vi "Connect.vi"(8 "error in":errorcluster, 11 "2727 in":refnum<class "2727.lvclass">) -> (0 "error out":errorcluster, 3 "2727 out":refnum<class "2727.lvclass">)   [LabVIEW 2019, in "2727.lvlib" / "2727.lvclass"]
uses:
  Library/2727.lvclass
  C:/Users/Public/Documents/Development/builds/Instruments/Instruments.lvlibp/Library/Instruments.lvclass
  Library/2727.lvclass/2727.ctl
  builds/Instruments/Instruments.lvlibp/Accessors/Read Resource.vi
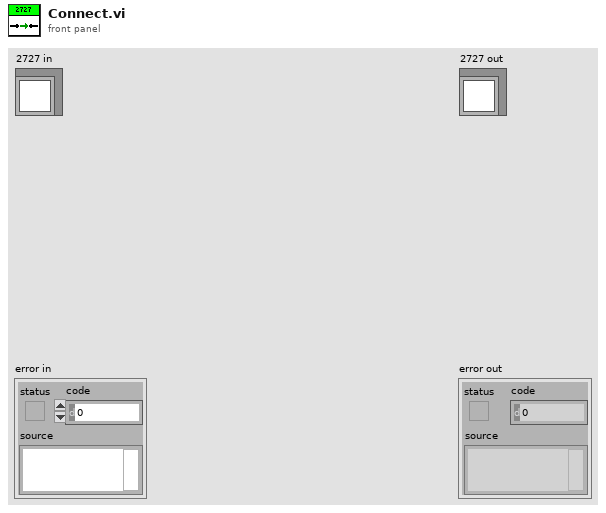
[diagram p1: front panel]
types:
  T1 = typedef "ni272x Reference.ctl" = refnum<k20>
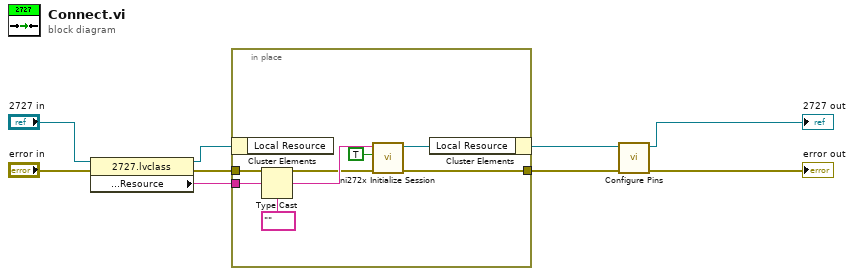
[diagram p0: block diagram]
diagram:
  n1 = property class="2727.lvclass"(reference="2727 in", error in="error in") -> (reference out=w6:refnum<class "2727.lvclass">, error out=w8:errorcluster, "Accessors:Configuration:Resource"=w5:string)
  n2 = in-place {
    in-place-border: w8 -> [w12]
    in-place-border: [w10] -> w3
    in-place-border: w5 -> [w15]
    n3 = in-place-cluster #1(w6) -> ()  [unwired: 1 out]
    n4 = Type Cast(type=tag "" ("*(type *) &x"), x=w15) -> (*(type *) &x=w13:tag)
    n5 = call <instrlib>:"ni272x Initialize Session.vi"("error in (no error)"=w12, "reset device (T)"=TRUE, "DAQmx Device Name"=w13) -> ("error out"=w10:errorcluster, "instrument handle out"=w11:T1)  [unwired: 7 out]
    n6 = in-place-cluster #1("Local Resource"=w11) -> (w4:refnum<class "2727.lvclass">)
  }
  n7 = call "Configure Pins.vi"("error in"=w3, "2727 in"=w4) -> ("error out"=→"error out":errorcluster, "2727 out"=→"2727 out":refnum<class "2727.lvclass">)  [unwired: 8 in]
